vi "FT_Get_Bit_Mode.vi"(0 "Handle":u32) -> (1 "FT_Status":u32(ring) items=["FT_OK", "FT_INVALID_HANDLE", "FT_DEVICE_NOT_FOUND", "FT_DEVICE_NOT_OPENED", "FT_IO_ERROR", "FT_INSUFFICIENT_RESOURCES", "FT_INVALID_PARAMETER", "FT_INVALID_BAUD_RATE", "FT_DEVICE_NOT_OPENED_FOR_ERASE", "FT_DEVICE_NOT_OPENED_FOR_WRITE", "FT_FAILED_TO_WRITE_DEVICE", "FT_EEPROM_READ_FAILED", "FT_EEPROM_WRITE_FAILED", "FT_EEPROM_ERASE_FAILED", "FT_EEPROM_NOT_PRESENT", "FT_EEPROM_NOT_PROGRAMMED", "FT_INVALID_ARGS", "FT_NOT_SUPPORTED", "FT_OTHER_ERROR"], 2 "Bit Mode":u8 format="%x", 3 "Pin States":T1)   [LabVIEW 2020]
uses:
  GEA3 DLL Source/ftd2xx.dll
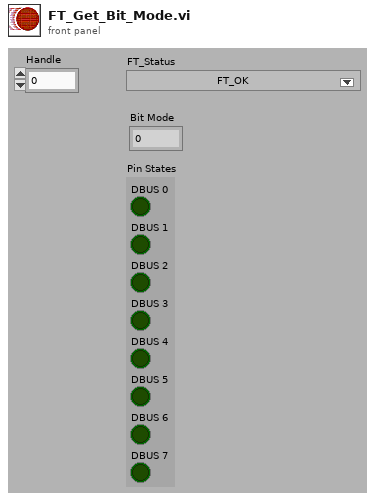
[diagram p1: front panel]
types:
  T1 = cluster{"DBUS 0":bool, "DBUS 1":bool, "DBUS 2":bool, "DBUS 3":bool, "DBUS 4":bool, "DBUS 5":bool, "DBUS 6":bool, "DBUS 7":bool}
  T2 = cluster{"Boolean array[0]":bool, "Boolean array[1]":bool, "Boolean array[2]":bool, "Boolean array[3]":bool, "Boolean array[4]":bool, "Boolean array[5]":bool, "Boolean array[6]":bool, "Boolean array[7]":bool}
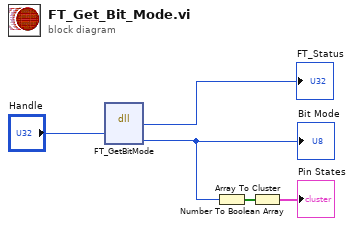
[diagram p0: block diagram]
diagram:
  n1 = dll-call lib="C:/TechnologyLab/NI-2010/Drivers/GEA3 Toolkit/GEA3 DLL Source/FTD2XX.dll" fn="FT_GetBitMode"("Handle"="Handle") -> ("FT_Status"=→"FT_Status":u32, "BitMode"=w2:u8)  [unwired: 5 in, 2 out]
  "Bit Mode" <- w2
  n2 = Number To Boolean Array(number=w2) -> (Boolean array=w3:bool[])
  n3 = Array To Cluster(array=w3) -> (cluster=→"Pin States":T2)
